vi "TPM with correction version 10-1-1 imaging.vi"() -> ()   [LabVIEW 2012]
uses:
  <vilib>/_Imagine Optic/VIs drivers/Data Haso/Wavefront parameters.ctl
  Program Files/Imagine Optic/Casao LabVIEW SDK/Casao/Casao/Loop prefs.ctl
  <vilib>/_Imagine Optic/VIs drivers/Data Haso/DataHaso.ctl
  <vilib>/Utility/file.llb/Read From Spreadsheet File (DBL).vi
  <vilib>/Utility/file.llb/Write To Spreadsheet File (DBL).vi
panel:
  in  "galvo phase":dbl=89.0
  out "output path":path
  out "Model Coefficients (µm) after":sgl[](array[numeric])
  out "Model Coefficients (µm) before":sgl[](array[numeric])
  in  "stop":bool
  out "Slice now":dbl
  in  "Iteration #":u16(ring)=1 items=["1"=1, "2"=2, "3"=3, "4"=4, "5"=5]
  in  "AO Exp Time":dbl(ring)=0.5 items=["0.2s"=0.2, "0.5s"=0.5, "1.0s"=1.0, "1.5s"=1.5]
  out "after correction":T1
  in  "Filter y tilt":bool=TRUE
  in  "Filter x tilt":bool=TRUE
  in  "Curvature filter":bool=TRUE
  out "PV":dbl
  out "RMS":dbl
  in  "Matrix path":path=path "C:/Documents and Settings/User/Desktop/zw/20160113 200nm bead command matrix.aomc"
  in  "Offset path":path=path "C:/Documents and Settings/User/Desktop/zw/2016-02-09 system resolution/100nm bead correction.dat"
  out "Camera image":u32[][](graph)
  out "RMS":dbl
  out "PV":dbl
  out "before correction":T1
  in  "Curvature filter":bool=TRUE
  in  "Filter y tilt":bool=TRUE
  in  "Filter x tilt":bool=TRUE
  out "after correction":dbl[][](graph) caption="Wavefront"
  out "before correction":dbl[][](graph) caption="Wavefront"
  in  "EMCCD ImExp Time (s)":dbl(ring)=0.5 items=["0.2"=0.2, "0.5"=0.5, "1.0"=1.0, "4.0"=4.0, "8.0"=8.0]
  in  "Step size(um)":dbl
  in  "Laser Power%(0-100)":dbl=10.0
  in  "Slices #":dbl=1.0
  in  "Average Frame #":dbl=10.0
  in  "Correction":bool
  # "OFF"
  # "ON"
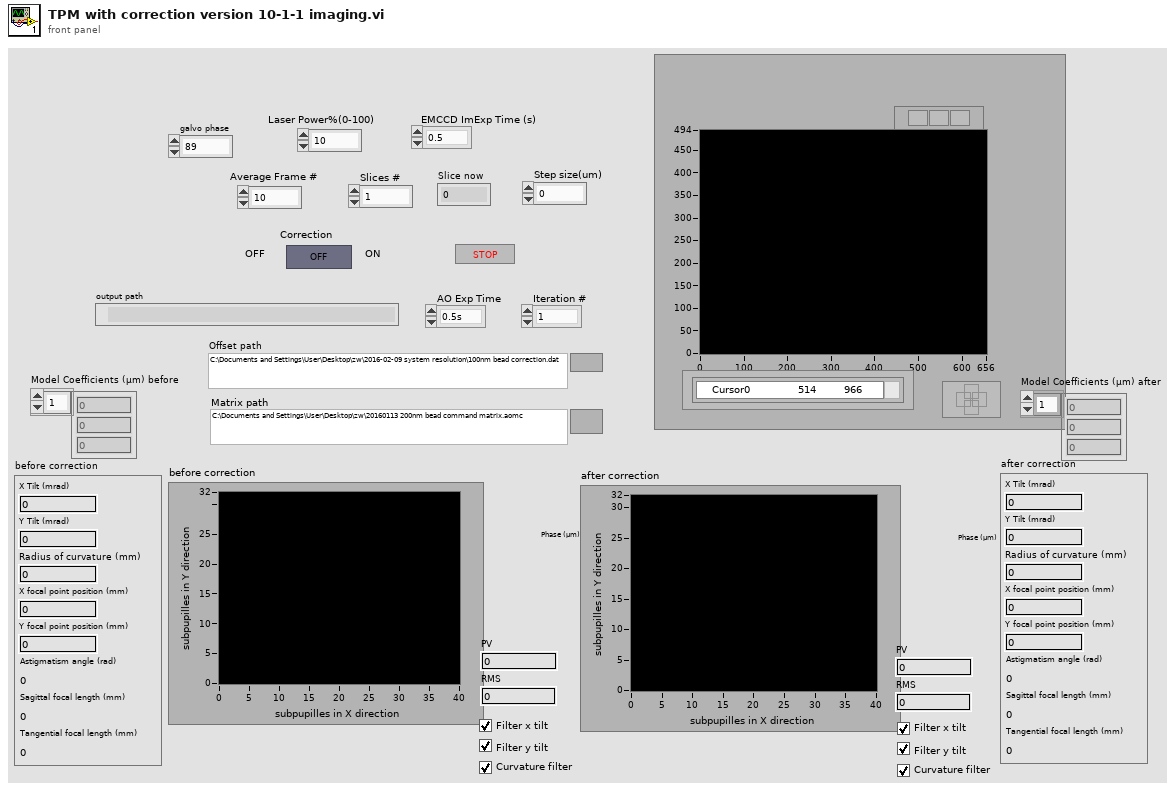
[diagram p1: front panel]
types:
  T1 = typedef "Wavefront parameters.ctl" = cluster{"X Tilt (mrad)":sgl, "Y Tilt (mrad)":sgl, "Radius of curvature (mm)":sgl, "X focal point position (mm)":sgl, "Y focal point position (mm)":sgl, "Astigmatism angle (rad)":sgl, "Sagittal focal length (mm)":sgl, "Tangential focal length (mm)":sgl}
  T2 = typedef "Loop prefs.ctl" = cluster{"Filter tilt on measurement (closed loop)":bool, "Correction gain (closed loop)":sgl, "Limit of subapertures off in CGP (%)":sgl, "Limit of saturated actuators (%)":sgl}
  T3 = cluster{"Filtre tilt X":bool, "Filtre tilt Y":bool, "Filtre courbure":bool}
  T4 = typedef "DataHaso.ctl" = i32
  T5 = cluster{"Measurement":T4, "Target":T4, "Manual target":T4}
  T6 = cluster{"Target for tilt":T4, "Target for focus":T4, "Target for all other aberrations":T4}
  T7 = typedef "Camera.ctl" = i32
  T8 = typedef "PhaseModul.ctl" = i32
  T9 = typedef "Haso.ctl" = i32
  T10 = typedef "Casao.ctl" = i32
  T11 = typedef "Image Compat.ctl" = cluster{"Signed/unsigned":bool, "Number of bits":T12, "Internal object id":i32, "Internal data id":i32}
  T12 = typedef "Data alignment enum.ctl" = enum16{"8", "16", "32"}
  T13 = typedef "Reconstruction prefs.ctl" = cluster{"Reconstruction type":enum16{"Modal", "Zonal"}, "Polynomial type":enum16{"Zernike", "Legendre"}, "Modal reconstruction prefs":T14, "Zonal reconstruction prefs":T17}
  T14 = typedef "Modal reconstruction prefs.ctl" = cluster{"Number of coefficients":u32, "Filtered coefficients":u32[], "RMS Zernike normalization":bool, "Matrix inversion method":u16, "Add zonal residual to modal fit ":bool, "Detection prefs":T15}
  T15 = typedef "PupilDetectionPrefs.ctl" = cluster{"Automatic pupil detection":bool, "Central occultation pupil":bool, "Semi-automatic pupil detection (find radius)":bool, "Semi-automatic pupil detection (find center)":bool, "Automatic pupil detection mode":enum16{"Contained", "Containing"}, "Start coordinates":cluster{"Pupil center (Zernike)":T16, "Pupil radius (Zernike)":sgl, "Pupil center (Legendre)":T16, "Pupil halfsize (Legendre)":T16}}
  T16 = typedef "Point2Df.ctl" = cluster{"X":sgl, "Y":sgl}
  T17 = typedef "Zonal reconstruction prefs.ctl" = cluster{"Number of weak iterations":u16, "Number of max iterations":u32, "Residual limit":sgl}
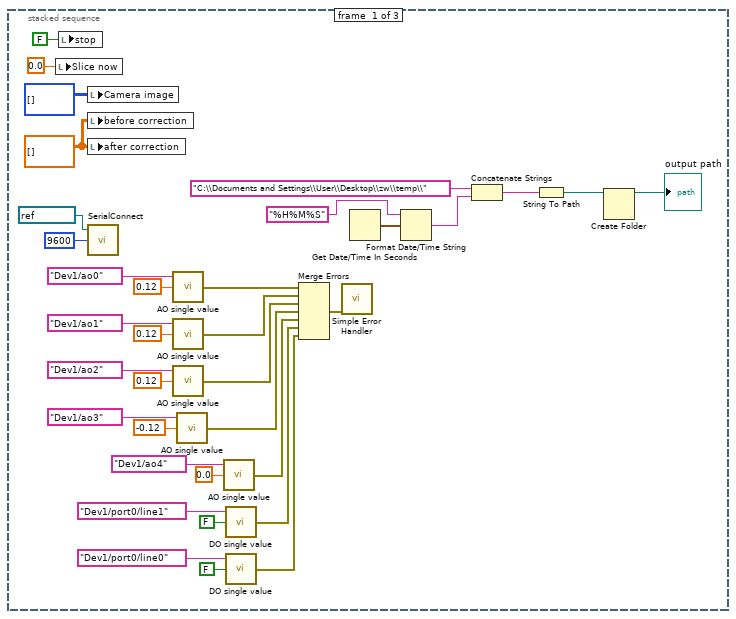
[diagram p2: hidden frame]
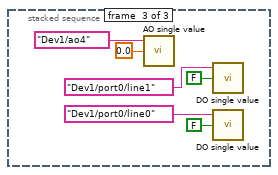
[diagram p10: hidden frame]
diagram:
  n1 = stacked-sequence {
    frame #0 {
      w34 = dbl[][] [] ("before correction")
      n2 = local write "Slice now"(0.0 ("Slice now")) -> ()
      n3 = local write "stop"(FALSE ("stop")) -> ()
      n4 = local write "Camera image"(u32[][] [] ("Camera image")) -> ()
      n5 = local write "before correction"(w34) -> ()
      n6 = local write "after correction"(w34) -> ()
      n7 = call "SerialConnect.vi"("baud rate (9600)"=u32 9600, "VISA resource name"=refnum<visa-resource-name> "COM1") -> ()  [unwired: 1 in, 3 out]
      n8 = call "AO single value.vi"("data"=0.12, "physical channels"=tag "Dev1/ao0") -> ("error out"=w17:errorcluster)  [unwired: 1 in]
      n9 = call "AO single value.vi"("data"=0.12, "physical channels"=tag "Dev1/ao1") -> ("error out"=w16:errorcluster)  [unwired: 1 in]
      n10 = call "AO single value.vi"("data"=0.12, "physical channels"=tag "Dev1/ao2") -> ("error out"=w15:errorcluster)  [unwired: 1 in]
      n11 = call "AO single value.vi"("data"=-0.12, "physical channels"=tag "Dev1/ao3") -> ("error out"=w14:errorcluster)  [unwired: 1 in]
      n12 = call "AO single value.vi"("data"=0.0, "physical channels"=tag "Dev1/ao4") -> ("error out"=w13:errorcluster)  [unwired: 1 in]
      n13 = call "DO single value.vi"("data"=FALSE, "lines"=tag "Dev1/port0/line1") -> ("error out"=w12:errorcluster)  [unwired: 1 in]
      n14 = call "DO single value.vi"("data"=FALSE, "lines"=tag "Dev1/port0/line0") -> ("error out"=w10:errorcluster)  [unwired: 1 in]
      n15 = Merge Errors(w17, w16, w15, w14, w13, w12, w10) -> (w11:errorcluster)
      n16 = call <vilib>:"Simple Error Handler.vi"("error in (no error)"=w11) -> ()  [unwired: 4 in, 5 out]
      n17 = Get Date/Time In Seconds() -> (seconds since 1Jan1904=w2:timestamp)
      n18 = Format Date/Time String(time format string (%c)="%H%M%S", seconds (now)=w2) -> (date/time string=w5:string)  [unwired: 1 in]
      n19 = Concatenate Strings("C:\\Documents and Settings\\User\\Desktop\\zw\\temp\\" ("string"), w5) -> (w6:string)
      n20 = String To Path(string=w6) -> (path=w7:path)
      n21 = Create Folder(path (use dialog)=w7) -> (created path=→"output path":path)  [unwired: 2 in, 2 out]
    }
    frame #1 {
      n22 = case shown="False" "Correction" {
        frame False {
          n23 = flat-sequence {
            frame #0 {
              n24 = call "DO single value.vi"("data"=TRUE, "lines"=tag "Dev1/port0/line1") -> ()  [unwired: 1 in, 1 out]
              n25 = call "DO single value.vi"("data"=FALSE, "lines"=tag "Dev1/port0/line0") -> ()  [unwired: 1 in, 1 out]
            }
            frame #1 {
              n26 = for {
                N: "Slices #" -> [_]
                i -> [w45]
                n27 = local read "stop"() -> (w43:bool)
                n28 = Not(x=w43) -> (.not. x?=w42:bool)
                n29 = Increment(x=w45) -> (x+1=w44:i32)
                n30 = case shown="True" w42 {
                  tunnel: w44 -> [_ w46]
                  frame False {
                  }
                  frame True {
                    n31 = flat-sequence {
                      frame #0 {
                        n32 = for {
                          N: "Average Frame #" -> [_]
                          n33 = local read "stop"() -> (w48:bool)
                          n34 = Not(x=w48) -> (.not. x?=w49:bool)
                          n35 = case shown="True" w49 {
                            frame False {
                            }
                            frame True {
                              n36 = flat-sequence {
                                tunnel: [w52] -> w50
                                tunnel: w50 -> [w74]
                                frame #0 {
                                n37 = local read "Laser Power%(0-100)"() -> (w63:dbl)
                                n38 = local read "EMCCD ImExp Time (s)"() -> (w62:dbl)
                                n39 = local read "galvo phase"() -> (w51:dbl)
                                n40 = call "waveform gen.vi"("Boolean"=TRUE, "galvo phase"=w51, "Exposure Time (s)"=w62, "Laser Power%(0-100)"=w63) -> ("waveform"=w60:waveform(dbl)[])
                                n41 = Index Array(array=w60, index=4) -> (element=w61:waveform(dbl))
                                n42 = call "AO triggle.vi"("physical channels"=tag "Dev1/ao0:4", "data"=w60, "waveform"=w61, "trig source"=tag "/Dev1/PFI1") -> ("task out"=w57:refnum<k21>, "error out"=w54:errorcluster)  [unwired: 1 in]
                                n43 = call "DO single value.vi"("error in"=w54, "data"=TRUE, "lines"=tag "Dev1/port0/line0") -> ("error out"=w53:errorcluster)
                                n44 = while {
                                tunnel: [w72] -> w66
                                tunnel: [w71] -> w65
                                tunnel: w57 -> [w69]
                                tunnel: w53 -> [w68]
                                stop <- w70 stop-if-true
                                n45 = call <vilib>:"DAQmx Is Task Done.vi"("task/channels in"=w69, "error in"=w68) -> ("task out"=w72:refnum<k21>, "task done?"=w70:bool, "error out"=w71:errorcluster)  [unwired: 11 in]
                                }
                                n46 = call <vilib>:"DAQmx Clear Task.vi"("task in"=w66, "error in"=w65) -> ("error out"=w52:errorcluster)  [unwired: 13 in]
                                }
                                frame #1 {
                                n47 = call "DO single value.vi"("error in"=w74, "data"=FALSE, "lines"=tag "Dev1/port0/line0") -> ("error out"=w73:errorcluster)
                                n48 = call "AO single value.vi"("error in"=w73, "data"=0.0, "physical channels"=tag "Dev1/ao4") -> ()  [unwired: 1 out]
                                }
                              }
                            }
                          }
                        }
                      }
                      frame #1 {
                        n49 = local read "Step size(um)"() -> (w79:dbl)
                        n50 = Multiply(x=w79, y=10.0) -> (x*y=w81:dbl)
                        n51 = Number To Decimal String(number=w81) -> (decimal integer string=w84:string)  [unwired: 1 in]
                        n52 = Concatenate Strings("movrel z=", w84) -> (w83:string)
                        n53 = call "WriteCmd.vi"("Command"=w83, "VISA resource name"=refnum<visa-resource-name> "COM1") -> ()  [unwired: 1 in, 1 out]
                      }
                      frame #2 {
                        n54 = Wait (ms)(milliseconds to wait=u32 50) -> ()  [unwired: 1 out]
                      }
                    }
                    n55 = local write "Slice now"(w46) -> ()
                  }
                }
              }
            }
            frame #2 {
            }
          }
        }
        frame True {
          n56 = flat-sequence {
            tunnel: [w102] -> w94
            tunnel: [w104] -> w93
            tunnel: [w103] -> w92
            tunnel: [w102] -> w91
            tunnel: [w101] -> w90
            tunnel: [w100] -> w88
            tunnel: [w95] -> w87
            tunnel: w94 -> [w123]
            tunnel: w93 -> [w122]
            tunnel: w92 -> [w121]
            tunnel: w91 -> [w118]
            tunnel: w90 -> [w117]
            tunnel: [w120] -> w89
            tunnel: w88 -> [w114]
            tunnel: w87 -> [w115]
            tunnel: w89 -> [w638]
            frame #0 {
              n57 = call "AO single value.vi"("data"=0.0, "physical channels"=tag "Dev1/ao4") -> ()  [unwired: 1 in, 1 out]
              n58 = local read "AO Exp Time"() -> (w105:dbl)
              n59 = call-poly <vilib>:"Read From Spreadsheet File.vi"("format (%.3f)"="%.8f", "file path (dialog if empty)"="Offset path") -> ("first row"=w95:dbl[])  [unwired: 5 in, 4 out]
              n60 = call "DO single value.vi"("data"=TRUE, "lines"=tag "Dev1/port0/line1") -> ()  [unwired: 1 in, 1 out]
              n61 = call "DO single value.vi"("data"=FALSE, "lines"=tag "Dev1/port0/line0") -> ()  [unwired: 1 in, 1 out]
              n62 = call "AO init.vi"("Exposure duration specified (s)"=w105, "Commands in"=w95, "Matrix path"="Matrix path") -> ("error out"=w102:errorcluster, "Camera"=w104:T7, "Mirror"=w100:T8, "Haso"=w103:T9, "Casao"=w101:T10)  [unwired: 3 in, 1 out]
            }
            frame #1 {
              n63 = call "Casao Set Preferences.vi"("error in (no error)"=w118, "Loop preferences"=T2 {"Filter tilt on measurement (closed loop)"=FALSE, "Correction gain (closed loop)"=0.75, "Limit of subapertures off in CGP (%)"=0.0, "Limit of saturated actuators (%)"=0.0}, "Casao"=w117) -> ("error out"=w112:errorcluster, "Casao (dup)"=w116:T10)  [unwired: 3 in]
              n64 = local read "Slices #"() -> (w124:dbl)
              n65 = call "PhaseModul apply command.vi"("error in (no error)"=w112, "Commands in"=w115, "Mirror"=w114) -> ("error out"=w111:errorcluster, "Mirror (dup)"=w113:T8)  [unwired: 2 in, 1 out]
              n66 = for {
                N: w124 -> [_]
                tunnel: w123 -> [w138]
                tunnel: w122 -> [w137]
                tunnel: w121 -> [w136]
                tunnel: w111 -> [w126]
                tunnel: [w135] -> w120
                tunnel: w113 -> [w127]
                tunnel: w116 -> [w134]
                tunnel: w115 -> [w125]
                i -> [w130]
                n67 = local read "stop"() -> (w132:bool)
                n68 = Increment(x=w130) -> (x+1=w133:i32)
                n69 = local write "Slice now"(w133) -> ()
                n70 = Not(x=w132) -> (.not. x?=w131:bool)
                n71 = case shown="True" w131 {
                  tunnel: w138 -> [_ w147]
                  tunnel: w137 -> [_ w146]
                  tunnel: w136 -> [_ w145]
                  tunnel: w126 -> [_ w144]
                  tunnel: [w139 w141] -> w135
                  tunnel: w127 -> [_ w143]
                  tunnel: w134 -> [w139 w142]
                  tunnel: w125 -> [_ w140]
                  frame False {
                  }
                  frame True {
                    n72 = flat-sequence {
                      tunnel: w147 -> [w187]
                      tunnel: w146 -> [w186]
                      tunnel: w145 -> [w185]
                      tunnel: w144 -> [w181]
                      tunnel: w143 -> [w172]
                      tunnel: w142 -> [w170]
                      tunnel: [w149] -> w141
                      tunnel: w140 -> [w148]
                      frame #0 {
                        n73 = flat-sequence {
                          tunnel: w170 -> [w190]
                          tunnel: w172 -> [w191]
                          tunnel: w181 -> [w192]
                          tunnel: w185 -> [w193]
                          tunnel: w186 -> [w194]
                          tunnel: w187 -> [w195]
                          tunnel: [w195] -> w155
                          tunnel: [w194] -> w154
                          tunnel: [w193] -> w153
                          tunnel: [w192] -> w152
                          tunnel: [w191] -> w151
                          tunnel: [w190] -> w150
                          tunnel: [w202] -> w161
                          tunnel: [w201] -> w160
                          tunnel: [w200] -> w159
                          tunnel: [w199] -> w158
                          tunnel: [w198] -> w157
                          tunnel: [w197] -> w156
                          tunnel: w155 -> [w202]
                          tunnel: w154 -> [w201]
                          tunnel: w153 -> [w200]
                          tunnel: w152 -> [w199]
                          tunnel: w151 -> [w198]
                          tunnel: w150 -> [w197]
                          tunnel: [w231] -> w184
                          tunnel: [w240] -> w183
                          tunnel: [w239] -> w182
                          tunnel: [w235] -> w180
                          tunnel: [w236] -> w179
                          tunnel: [w233] -> w173
                          tunnel: w161 -> [w232]
                          tunnel: w160 -> [w240]
                          tunnel: w159 -> [w239]
                          tunnel: w158 -> [w236]
                          tunnel: w157 -> [w234]
                          tunnel: w156 -> [w235]
                          tunnel: w148 -> [w230]
                          tunnel: w184 -> [w282]
                          tunnel: w183 -> [w281]
                          tunnel: w182 -> [w280]
                          tunnel: w180 -> [w279]
                          tunnel: w179 -> [w278]
                          tunnel: [w258] -> w178
                          tunnel: [w257] -> w177
                          tunnel: [w253] -> w176
                          tunnel: [w251] -> w175
                          tunnel: [w249] -> w174
                          tunnel: w173 -> [w244]
                          tunnel: [w243] -> w171
                          tunnel: [w241] -> w163
                          tunnel: w178 -> [w424]
                          tunnel: w177 -> [w423]
                          tunnel: w176 -> [w421]
                          tunnel: w175 -> [w420]
                          tunnel: w174 -> [w419]
                          tunnel: [w418] -> w169
                          tunnel: w171 -> [w417]
                          tunnel: [w416] -> w168
                          tunnel: [w415] -> w167
                          tunnel: [w414] -> w166
                          tunnel: [w413] -> w165
                          tunnel: [w412] -> w164
                          tunnel: w163 -> [w411]
                          tunnel: [w411] -> w162
                          tunnel: w169 -> [w603]
                          tunnel: w168 -> [w622]
                          tunnel: w167 -> [w621]
                          tunnel: w166 -> [w620]
                          tunnel: w165 -> [w610]
                          tunnel: w164 -> [w611]
                          tunnel: w162 -> [w609]
                          tunnel: [w603] -> w149
                          frame #0 {
                            n74 = call "AO single value.vi"("data"=-5.0, "physical channels"=tag "Dev1/ao5") -> ()  [unwired: 1 in, 1 out]
                          }
                          frame #1 {
                            n75 = local read "Average Frame #"() -> (w196:dbl)
                            n76 = for {
                              N: w196 -> [_]
                              n77 = local read "stop"() -> (w203:bool)
                              n78 = Not(x=w203) -> (.not. x?=w204:bool)
                              n79 = case shown="True" w204 {
                                frame False {
                                }
                                frame True {
                                n80 = flat-sequence {
                                frame #0 {
                                n81 = local read "Laser Power%(0-100)"() -> (w216:dbl)
                                n82 = local read "EMCCD ImExp Time (s)"() -> (w215:dbl)
                                n83 = call "waveform gen.vi"("Boolean"=TRUE, "galvo phase"="galvo phase", "Exposure Time (s)"=w215, "Laser Power%(0-100)"=w216) -> ("waveform"=w213:waveform(dbl)[])
                                n84 = Index Array(array=w213, index=4) -> (element=w214:waveform(dbl))
                                n85 = call "AO triggle.vi"("physical channels"=tag "Dev1/ao0:4", "data"=w213, "waveform"=w214, "trig source"=tag "/Dev1/PFI0") -> ("task out"=w210:refnum<k21>, "error out"=w207:errorcluster)  [unwired: 1 in]
                                n86 = call "DO single value.vi"("error in"=w207, "data"=TRUE, "lines"=tag "Dev1/port0/line0") -> ("error out"=w206:errorcluster)
                                n87 = while {
                                tunnel: [w225] -> w219
                                tunnel: [w224] -> w218
                                tunnel: w210 -> [w222]
                                tunnel: w206 -> [w221]
                                stop <- w223 stop-if-true
                                n88 = call <vilib>:"DAQmx Is Task Done.vi"("task/channels in"=w222, "error in"=w221) -> ("task out"=w225:refnum<k21>, "task done?"=w223:bool, "error out"=w224:errorcluster)  [unwired: 11 in]
                                }
                                n89 = call <vilib>:"DAQmx Clear Task.vi"("task in"=w219, "error in"=w218) -> ()  [unwired: 13 in, 1 out]
                                }
                                frame #1 {
                                n90 = call "AO single value.vi"("data"=0.0, "physical channels"=tag "Dev1/ao4") -> ()  [unwired: 1 in, 1 out]
                                n91 = call "DO single value.vi"("data"=FALSE, "lines"=tag "Dev1/port0/line0") -> ()  [unwired: 1 in, 1 out]
                                }
                                }
                                }
                              }
                            }
                          }
                          frame #2 {
                            n92 = call "PhaseModul apply command.vi"("error in (no error)"=w232, "Commands in"=w230, "Mirror"=w234) -> ("error out"=w231:errorcluster, "Mirror (dup)"=w233:T8)  [unwired: 2 in, 1 out]
                            n93 = call "AO single value.vi"("data"=1.0, "physical channels"=tag "Dev1/ao5") -> ()  [unwired: 1 in, 1 out]
                          }
                          frame #3 {
                            n94 = flat-sequence {
                              tunnel: [w291] -> w277
                              tunnel: [w290] -> w276
                              tunnel: [w289] -> w275
                              tunnel: [w288] -> w274
                              tunnel: [w287] -> w273
                              tunnel: w280 -> [w289]
                              tunnel: w281 -> [w290]
                              tunnel: w282 -> [w291]
                              tunnel: [w286] -> w272
                              tunnel: w279 -> [w286]
                              tunnel: [w285] -> w271
                              tunnel: w278 -> [w285]
                              tunnel: [w284] -> w245
                              tunnel: w244 -> [w284]
                              tunnel: w277 -> [w307]
                              tunnel: w276 -> [w308]
                              tunnel: w275 -> [w309]
                              tunnel: [w309] -> w270
                              tunnel: [w306] -> w269
                              tunnel: [w305] -> w268
                              tunnel: [w304] -> w267
                              tunnel: w274 -> [w304]
                              tunnel: [w303] -> w266
                              tunnel: w273 -> [w303]
                              tunnel: [w302] -> w265
                              tunnel: w272 -> [w302]
                              tunnel: [w301] -> w264
                              tunnel: w271 -> [w301]
                              tunnel: [w300] -> w246
                              tunnel: w245 -> [w300]
                              tunnel: w270 -> [w321]
                              tunnel: [w321] -> w261
                              tunnel: [w320] -> w262
                              tunnel: w269 -> [w320]
                              tunnel: [w319] -> w263
                              tunnel: w268 -> [w319]
                              tunnel: w267 -> [w314]
                              tunnel: w266 -> [w313]
                              tunnel: [w312] -> w260
                              tunnel: w265 -> [w312]
                              tunnel: [w311] -> w259
                              tunnel: w264 -> [w311]
                              tunnel: [w310] -> w247
                              tunnel: w246 -> [w310]
                              tunnel: w263 -> [w403]
                              tunnel: w262 -> [w363]
                              tunnel: w261 -> [w364]
                              tunnel: w260 -> [w389]
                              tunnel: w259 -> [w388]
                              tunnel: [w367] -> w256
                              tunnel: [w366] -> w255
                              tunnel: [w365] -> w254
                              tunnel: [w364] -> w252
                              tunnel: [w363] -> w250
                              tunnel: [w362] -> w248
                              tunnel: w247 -> [w361]
                              tunnel: [w361] -> w242
                              tunnel: [w335] -> w241
                              tunnel: [w409] -> w257
                              tunnel: [w410] -> w258
                              tunnel: w256 -> [w410]
                              tunnel: w255 -> [w409]
                              tunnel: w254 -> [w408]
                              tunnel: [w407] -> w253
                              tunnel: w252 -> [w407]
                              tunnel: [w406] -> w251
                              tunnel: w250 -> [w406]
                              tunnel: [w405] -> w249
                              tunnel: w248 -> [w405]
                              tunnel: [w404] -> w243
                              tunnel: w242 -> [w404]
                              frame #0 {
                                n95 = local read "Laser Power%(0-100)"() -> (w297:dbl)
                                n96 = local read "AO Exp Time"() -> (w296:dbl)
                                n97 = local read "galvo phase"() -> (w283:dbl)
                                n98 = call "waveform gen.vi"("Boolean"=FALSE, "galvo phase"=w283, "Exposure Time (s)"=w296, "Laser Power%(0-100)"=w297) -> ("waveform"=w295:waveform(dbl)[])
                                n99 = Index Array(array=w295, index=4) -> (element=w294:waveform(dbl))
                                n100 = call "AO triggle.vi"("physical channels"=tag "Dev1/ao0:4", "data"=w295, "waveform"=w294, "trig source"=tag "/Dev1/PFI1") -> ("task out"=w288:refnum<k21>, "error out"=w287:errorcluster)  [unwired: 1 in]
                              }
                              frame #1 {
                                n101 = call <vilib>:"Camera Start.vi"("error in (no error)"=w307, "camera"=w308) -> ("error out"=w305:errorcluster, "camera (dup)"=w306:T7)  [unwired: 4 in]
                              }
                              frame #2 {
                                n102 = while {
                                tunnel: [w326] -> w316
                                tunnel: [w325] -> w315
                                tunnel: w314 -> [w323]
                                tunnel: w313 -> [w322]
                                stop <- w324 stop-if-true
                                n103 = call <vilib>:"DAQmx Is Task Done.vi"("task/channels in"=w323, "error in"=w322) -> ("task out"=w326:refnum<k21>, "task done?"=w324:bool, "error out"=w325:errorcluster)  [unwired: 11 in]
                                }
                                n104 = call "DO single value.vi"("data"=TRUE, "lines"=tag "Dev1/port0/line0") -> ()  [unwired: 1 in, 1 out]
                                n105 = call <vilib>:"DAQmx Clear Task.vi"("task in"=w316, "error in"=w315) -> ()  [unwired: 13 in, 1 out]
                              }
                              frame #3 {
                                n106 = call <vilib>:"Camera Get image.vi"("error in (no error)"=w403, "camera"=w363) -> ("error out"=w385:errorcluster, "Image"=w386:T11, "camera (dup)"=w387:T7)  [unwired: 3 in]
                                n107 = call <vilib>:"Camera Stop.vi"("error in (no error)"=w385, "camera"=w387) -> ()  [unwired: 4 in, 2 out]
                                n108 = call "Image get data.vi"("error in (no error)"=w385, "Image Compat"=w386) -> ("error out"=w375:errorcluster, "Array"=w384:u32[][], "Image Compat (dup)"=w374:T11)  [unwired: 3 in]
                                n109 = call "AO single value.vi"("data"=0.0, "physical channels"=tag "Dev1/ao4") -> ()  [unwired: 1 in, 1 out]
                                n110 = local write "Camera image"(w384) -> ()
                                n111 = call <vilib>:"Haso compute slopes.vi"("error in (no error)"=w375, "Image Compat"=w374, "Haso"=w364) -> ("error out"=w333:errorcluster, "Data Haso"=w337:T4)  [unwired: 1 in, 2 out]
                                n112 = call "DO single value.vi"("data"=FALSE, "lines"=tag "Dev1/port0/line0") -> ()  [unwired: 1 in, 1 out]
                                n113 = call "DataHaso ctor copie.vi"("error in (no error)"=w333, "DataHaso"=w337) -> ("error out"=w332:errorcluster, "new DataHaso"=w335:T4, "DataHaso (dup)"=w334:T4)  [unwired: 3 in]
                                n114 = call "DataHaso get reconstruction prefs.vi"("error in (no error)"=w332, "Data Haso"=w334) -> ("error out"=w348:errorcluster, "Reconstruction Preferences"=w344:T13, "Data Haso (dup)"=w347:T4)  [unwired: 3 in]
                                n115 = Bundle By Name(cluster=w344, "Reconstruction type"=enum16{"Modal", "Zonal"}."Modal", "Polynomial type"=enum16{"Zernike", "Legendre"}."Zernike", "Modal reconstruction prefs.Number of coefficients"=u32 32) -> (w343:T13)
                                n116 = call <vilib>:"DataHaso set reconstruction prefs.vi"("error in (no error)"=w348, "Reconstruction Preferences"=w343, "Data Haso"=w347) -> ("error out"=w345:errorcluster, "Data Haso (dup)"=w346:T4)  [unwired: 3 in]
                                n117 = call "DataHaso get modal coefficients.vi"("error in (no error)"=w345, "Data Haso"=w346) -> ("error out"=w338:errorcluster, "Coefficients (µm)"=w349:sgl[], "Data Haso (dup)"=w339:T4)  [unwired: 3 in]
                                "Model Coefficients (µm) before" <- w349
                                n118 = Bundle By Name(cluster=T3 {"Filtre tilt X"=FALSE, "Filtre tilt Y"=FALSE, "Filtre courbure"=FALSE} ("Filtre"), "Filtre tilt X"="Filter x tilt", "Filtre tilt Y"="Filter y tilt", "Filtre courbure"="Curvature filter") -> (w369:T3)
                                n119 = call <vilib>:"DataHaso parameters.vi"("error in (no error)"=w338, "Data Haso"=w339) -> ("error out"=w382:errorcluster, "Parameters"=w357:T1, "Data Haso (dup)"=w383:T4)  [unwired: 3 in]
                                "before correction" <- w357
                                n120 = control-ref of="before correction"() -> (w368:refnum<vi>)
                                n121 = call "DataHaso filter tilt or curvature.vi"("error in (no error)"=w382, "Filter (default: all true)"=w369, "Data Haso"=w383) -> ("error out"=w380:errorcluster, "Data Haso (dup)"=w381:T4)  [unwired: 3 in]
                                n122 = local read "Slice now"() -> (w351:dbl)
                                n123 = call "DataHaso phase.vi"("error in (no error)"=w380, "Data Haso"=w381) -> ("error out"=w378:errorcluster, "Phase (µm)"=w379:i32, "Data Haso (dup)"=w336:T4)  [unwired: 3 in]
                                n124 = Number To Decimal String(number=w351) -> (decimal integer string=w353:string)  [unwired: 1 in]
                                n125 = call "Formatter Intensity Graph.vi"("error in (no error)"=w378, "Intensity Graph"=w368, "Surface with pupil"=w379) -> ("error out"=w376:errorcluster, "Surface with pupil (dup)"=w377:i32)  [unwired: 2 in, 1 out]
                                n126 = call <vilib>:"Surface with pupil get stats.vi"("error in (no error)"=w376, "Surface Avec Pupille"=w377) -> ("error out"=w362:errorcluster, "PV"=w360:sgl, "RMS"=w359:dbl)  [unwired: 2 in, 1 out]
                                "PV" <- w360
                                "RMS" <- w359
                                n127 = local read "output path"() -> (w327:path)
                                n128 = Concatenate Strings("before_slice", w353, ".dat") -> (w328:string)
                                n129 = Cluster To Array(cluster=w357) -> (array=w358:sgl[])
                                n130 = Build Path(base path=w327, name or relative path=w328) -> (appended path=w329:path)
                                n131 = Build Array (concatenate)(w360, w359, w358, w349) -> (w356:dbl[])
                                n132 = Merge Errors(w362, w388) -> (w398:errorcluster)
                                n133 = Bundle By Name(cluster=T6 {"Target for tilt"=0, "Target for focus"=0, "Target for all other aberrations"=0} ("References"), "Target for tilt"=w335, "Target for focus"=w335) -> (w401:T6)
                                n134 = call "DataHaso ctor copie.vi"("error in (no error)"=w398, "DataHaso"=w336) -> ("error out"=w400:errorcluster, "new DataHaso"=w399:T4)  [unwired: 3 in, 1 out]
                                n135 = call-poly <vilib>:"Write To Spreadsheet File.vi"("transpose? (no:F)"=TRUE, "format (%.3f)"="%.6f", "1D data"=w356, "file path (dialog if empty)"=w329) -> ()  [unwired: 4 in, 1 out]
                                n136 = call "Casao Compute target.vi"("error in (no error)"=w400, "Targets"=w401, "DataHaso"=w399, "Casao"=w389) -> ("error out"=w396:errorcluster, "DataHaso (dup)"=w365:T4, "Casao (dup)"=w397:T10)  [unwired: 1 out]
                                n137 = Bundle By Name(cluster=T5 {"Measurement"=0, "Target"=0, "Manual target"=0} ("Slopes"), "Measurement"=w336, "Target"=w365) -> (w395:T5)
                                n138 = call "Casao get correction commands.vi"("Casao"=w397, "Slopes"=w395, "error in (no error)"=w396) -> ("Casao (dup)"=w367:T10, "Commands"=w392:sgl[], "error out"=w393:errorcluster)  [unwired: 2 in, 2 out]
                                n139 = call "PhaseModul apply command.vi"("error in (no error)"=w393, "Commands in"=w392, "Mirror"=w361) -> ("error out"=w366:errorcluster)  [unwired: 2 in, 2 out]
                              }
                              frame #4 {
                                n140 = call "DataHaso dtor.vi"("Data Haso"=w408) -> ()  [unwired: 6 in, 1 out]
                              }
                            }
                          }
                          frame #4 {
                            n141 = for {
                              N: "Iteration #" -> [_]
                              tunnel: w424 -> [w453]
                              tunnel: w423 -> [w452]
                              tunnel: w421 -> [w451]
                              tunnel: w420 -> [w450]
                              tunnel: w419 -> [w449]
                              tunnel: [w447] -> w418
                              tunnel: w417 -> [w442]
                              tunnel: [w441] -> w416
                              tunnel: [w439] -> w415
                              tunnel: [w437] -> w414
                              tunnel: [w435] -> w413
                              tunnel: [w432] -> w412
                              tunnel: w411 -> [w431]
                              i -> [w430]
                              n142 = Increment(x=w430) -> (x+1=w429:i32)
                              n143 = flat-sequence {
                                tunnel: [w478] -> w472
                                tunnel: [w479] -> w471
                                tunnel: [w480] -> w470
                                tunnel: [w484] -> w469
                                tunnel: [w483] -> w468
                                tunnel: [w482] -> w467
                                tunnel: [w481] -> w466
                                tunnel: w453 -> [w482]
                                tunnel: w452 -> [w481]
                                tunnel: w451 -> [w480]
                                tunnel: w450 -> [w479]
                                tunnel: w449 -> [w478]
                                tunnel: [w477] -> w443
                                tunnel: w442 -> [w477]
                                tunnel: w429 -> [w475]
                                tunnel: [w474] -> w426
                                tunnel: w472 -> [w501]
                                tunnel: w471 -> [w502]
                                tunnel: w470 -> [w503]
                                tunnel: [w503] -> w465
                                tunnel: [w500] -> w464
                                tunnel: [w499] -> w463
                                tunnel: [w498] -> w462
                                tunnel: w469 -> [w498]
                                tunnel: [w497] -> w461
                                tunnel: w468 -> [w497]
                                tunnel: [w496] -> w460
                                tunnel: w467 -> [w496]
                                tunnel: [w495] -> w459
                                tunnel: w466 -> [w495]
                                tunnel: [w494] -> w444
                                tunnel: w443 -> [w494]
                                tunnel: [w493] -> w427
                                tunnel: w426 -> [w493]
                                tunnel: w465 -> [w516]
                                tunnel: [w516] -> w456
                                tunnel: [w515] -> w457
                                tunnel: w464 -> [w515]
                                tunnel: [w514] -> w458
                                tunnel: w463 -> [w514]
                                tunnel: w462 -> [w509]
                                tunnel: w461 -> [w508]
                                tunnel: [w507] -> w455
                                tunnel: w460 -> [w507]
                                tunnel: [w506] -> w454
                                tunnel: w459 -> [w506]
                                tunnel: [w505] -> w445
                                tunnel: w444 -> [w505]
                                tunnel: [w504] -> w428
                                tunnel: w427 -> [w504]
                                tunnel: w458 -> [w584]
                                tunnel: w457 -> [w585]
                                tunnel: w456 -> [w586]
                                tunnel: w455 -> [w571]
                                tunnel: w454 -> [w570]
                                tunnel: [w550] -> w448
                                tunnel: [w549] -> w446
                                tunnel: w445 -> [w529]
                                tunnel: [w545] -> w440
                                tunnel: [w544] -> w438
                                tunnel: [w543] -> w436
                                tunnel: [w542] -> w434
                                tunnel: [w531] -> w433
                                tunnel: w431 -> [w528]
                                tunnel: w428 -> [w525]
                                tunnel: [w522] -> w425
                                tunnel: w448 -> [w598]
                                tunnel: [w597] -> w447
                                tunnel: w446 -> [w597]
                                tunnel: [w596] -> w441
                                tunnel: w440 -> [w596]
                                tunnel: [w595] -> w439
                                tunnel: w438 -> [w595]
                                tunnel: [w594] -> w437
                                tunnel: w436 -> [w594]
                                tunnel: [w590] -> w435
                                tunnel: w434 -> [w591]
                                tunnel: w433 -> [w593]
                                tunnel: [w593] -> w432
                                tunnel: w425 -> [w592]
                                frame #0 {
                                n144 = local read "Laser Power%(0-100)"() -> (w490:dbl)
                                n145 = local read "AO Exp Time"() -> (w489:dbl)
                                n146 = local read "galvo phase"() -> (w473:dbl)
                                n147 = call "waveform gen.vi"("Boolean"=FALSE, "galvo phase"=w473, "Exposure Time (s)"=w489, "Laser Power%(0-100)"=w490) -> ("waveform"=w488:waveform(dbl)[])
                                n148 = local read "Iteration #"() -> (w476:u16)
                                n149 = Index Array(array=w488, index=4) -> (element=w487:waveform(dbl))
                                n150 = Less?(x=w476, y=w475) -> (x < y?=w474:bool)
                                n151 = call "AO triggle.vi"("physical channels"=tag "Dev1/ao0:4", "data"=w488, "waveform"=w487, "trig source"=tag "/Dev1/PFI1") -> ("task out"=w484:refnum<k21>, "error out"=w483:errorcluster)  [unwired: 1 in]
                                }
                                frame #1 {
                                n152 = call <vilib>:"Camera Start.vi"("error in (no error)"=w501, "camera"=w502) -> ("error out"=w499:errorcluster, "camera (dup)"=w500:T7)  [unwired: 4 in]
                                }
                                frame #2 {
                                n153 = while {
                                tunnel: [w521] -> w511
                                tunnel: [w520] -> w510
                                tunnel: w509 -> [w518]
                                tunnel: w508 -> [w517]
                                stop <- w519 stop-if-true
                                n154 = call <vilib>:"DAQmx Is Task Done.vi"("task/channels in"=w518, "error in"=w517) -> ("task out"=w521:refnum<k21>, "task done?"=w519:bool, "error out"=w520:errorcluster)  [unwired: 11 in]
                                }
                                n155 = call "DO single value.vi"("data"=TRUE, "lines"=tag "Dev1/port0/line0") -> ()  [unwired: 1 in, 1 out]
                                n156 = call <vilib>:"DAQmx Clear Task.vi"("task in"=w511, "error in"=w510) -> ()  [unwired: 13 in, 1 out]
                                }
                                frame #3 {
                                n157 = call <vilib>:"Camera Get image.vi"("error in (no error)"=w584, "camera"=w585) -> ("error out"=w567:errorcluster, "Image"=w568:T11, "camera (dup)"=w569:T7)  [unwired: 3 in]
                                n158 = call <vilib>:"Camera Stop.vi"("error in (no error)"=w567, "camera"=w569) -> ()  [unwired: 4 in, 2 out]
                                n159 = call "Image get data.vi"("error in (no error)"=w567, "Image Compat"=w568) -> ("error out"=w557:errorcluster, "Array"=w566:u32[][], "Image Compat (dup)"=w556:T11)  [unwired: 3 in]
                                n160 = call "AO single value.vi"("data"=0.0, "physical channels"=tag "Dev1/ao4") -> ()  [unwired: 1 in, 1 out]
                                n161 = local write "Camera image"(w566) -> ()
                                n162 = call <vilib>:"Haso compute slopes.vi"("error in (no error)"=w557, "Image Compat"=w556, "Haso"=w586) -> ("error out"=w534:errorcluster, "Data Haso"=w533:T4)  [unwired: 1 in, 2 out]
                                n163 = call "DO single value.vi"("data"=FALSE, "lines"=tag "Dev1/port0/line0") -> ()  [unwired: 1 in, 1 out]
                                n164 = call "DataHaso get reconstruction prefs.vi"("error in (no error)"=w534, "Data Haso"=w533) -> ("error out"=w540:errorcluster, "Reconstruction Preferences"=w539:T13, "Data Haso (dup)"=w541:T4)  [unwired: 3 in]
                                n165 = Bundle By Name(cluster=w539, "Reconstruction type"=enum16{"Modal", "Zonal"}."Modal", "Polynomial type"=enum16{"Zernike", "Legendre"}."Zernike", "Modal reconstruction prefs.Number of coefficients"=u32 32) -> (w538:T13)
                                n166 = call <vilib>:"DataHaso set reconstruction prefs.vi"("error in (no error)"=w540, "Reconstruction Preferences"=w538, "Data Haso"=w541) -> ("error out"=w526:errorcluster, "Data Haso (dup)"=w527:T4)  [unwired: 3 in]
                                n167 = call "DataHaso get modal coefficients.vi"("error in (no error)"=w526, "Data Haso"=w527) -> ("error out"=w532:errorcluster, "Coefficients (µm)"=w531:sgl[], "Data Haso (dup)"=w530:T4)  [unwired: 3 in]
                                "Model Coefficients (µm) after" <- w531
                                n168 = Bundle By Name(cluster=T3 {"Filtre tilt X"=FALSE, "Filtre tilt Y"=FALSE, "Filtre courbure"=FALSE} ("Filtre"), "Filtre tilt X"="Filter x tilt", "Filtre tilt Y"="Filter y tilt", "Filtre courbure"="Curvature filter") -> (w554:T3)
                                n169 = call <vilib>:"DataHaso parameters.vi"("error in (no error)"=w532, "Data Haso"=w530) -> ("error out"=w564:errorcluster, "Parameters"=w543:T1, "Data Haso (dup)"=w565:T4)  [unwired: 3 in]
                                "after correction" <- w543
                                n170 = control-ref of="after correction"() -> (w548:refnum<vi>)
                                n171 = call "DataHaso filter tilt or curvature.vi"("error in (no error)"=w564, "Filter (default: all true)"=w554, "Data Haso"=w565) -> ("error out"=w562:errorcluster, "Data Haso (dup)"=w563:T4)  [unwired: 3 in]
                                n172 = call "DataHaso phase.vi"("error in (no error)"=w562, "Data Haso"=w563) -> ("error out"=w560:errorcluster, "Phase (µm)"=w561:i32, "Data Haso (dup)"=w547:T4)  [unwired: 3 in]
                                n173 = call "Formatter Intensity Graph.vi"("error in (no error)"=w560, "Intensity Graph"=w548, "Surface with pupil"=w561) -> ("error out"=w558:errorcluster, "Surface with pupil (dup)"=w559:i32)  [unwired: 2 in, 1 out]
                                n174 = call <vilib>:"Surface with pupil get stats.vi"("error in (no error)"=w558, "Surface Avec Pupille"=w559) -> ("error out"=w579:errorcluster, "PV"=w544:sgl, "RMS"=w545:dbl)  [unwired: 2 in, 1 out]
                                "RMS" <- w545
                                "PV" <- w544
                                n175 = Merge Errors(w579, w570) -> (w578:errorcluster)
                                n176 = Bundle By Name(cluster=T6 {"Target for tilt"=0, "Target for focus"=0, "Target for all other aberrations"=0} ("References"), "Target for tilt"=w528, "Target for focus"=w528) -> (w582:T6)
                                n177 = call "DataHaso ctor copie.vi"("error in (no error)"=w578, "DataHaso"=w547) -> ("error out"=w581:errorcluster, "new DataHaso"=w580:T4, "DataHaso (dup)"=w546:T4)  [unwired: 3 in]
                                n178 = call "Casao Compute target.vi"("error in (no error)"=w581, "Targets"=w582, "DataHaso"=w580, "Casao"=w571) -> ("error out"=w576:errorcluster, "DataHaso (dup)"=w550:T4, "Casao (dup)"=w577:T10)  [unwired: 1 out]
                                n179 = Bundle By Name(cluster=T5 {"Measurement"=0, "Target"=0, "Manual target"=0} ("Slopes"), "Measurement"=w546, "Target"=w550) -> (w575:T5)
                                n180 = call "Casao get correction commands.vi"("Casao"=w577, "Slopes"=w575, "error in (no error)"=w576) -> ("Casao (dup)"=w549:T10, "Commands"=w542:sgl[], "error out"=w522:errorcluster)  [unwired: 2 in, 2 out]
                                n181 = case shown="True" w525 {
                                tunnel: w522 -> [_ w589]
                                tunnel: w542 -> [_ w588]
                                tunnel: w529 -> [_ w587]
                                frame False {
                                }
                                frame True {
                                n182 = call "PhaseModul apply command.vi"("error in (no error)"=w589, "Commands in"=w588, "Mirror"=w587) -> ()  [unwired: 2 in, 3 out]
                                }
                                }
                                }
                                frame #4 {
                                n183 = call "DataHaso dtor.vi"("Data Haso"=w598) -> ()  [unwired: 6 in, 1 out]
                                n184 = case shown="Error" w592 {
                                tunnel: w591 -> [w599 _]
                                tunnel: [w599 w600] -> w590
                                frame No Error {
                                }
                                frame Error {
                                n185 = Initialize Array(0.0 ("element"), 52 ("dimension size")) -> (w600:dbl[])
                                }
                                }
                                }
                              }
                            }
                          }
                          frame #5 {
                            n186 = call "DataHaso dtor.vi"("Data Haso"=w609) -> ()  [unwired: 6 in, 1 out]
                            n187 = local read "Slice now"() -> (w614:dbl)
                            n188 = Cluster To Array(cluster=w620) -> (array=w619:sgl[])
                            n189 = Build Array (concatenate)(w621, w622, w619, w611) -> (w627:dbl[])
                            n190 = Number To Decimal String(number=w614) -> (decimal integer string=w624:string)  [unwired: 1 in]
                            n191 = Number To Decimal String(number=w614) -> (decimal integer string=w616:string)  [unwired: 1 in]
                            n192 = call "AO single value.vi"("data"=0.0, "physical channels"=tag "Dev1/ao4") -> ()  [unwired: 1 in, 1 out]
                            n193 = local read "output path"() -> (w604:path)
                            n194 = Concatenate Strings("afterC_slice", w624, ".dat") -> (w608:string)
                            n195 = Concatenate Strings("command", w616, ".dat") -> (w605:string)
                            n196 = Build Path(base path=w604, name or relative path=w608) -> (appended path=w607:path)
                            n197 = Build Path(base path=w604, name or relative path=w605) -> (appended path=w606:path)
                            n198 = call-poly <vilib>:"Write To Spreadsheet File.vi"("transpose? (no:F)"=TRUE, "format (%.3f)"="%.6f", "1D data"=w627, "file path (dialog if empty)"=w607) -> ()  [unwired: 4 in, 1 out]
                            n199 = call-poly <vilib>:"Write To Spreadsheet File.vi"("transpose? (no:F)"=TRUE, "format (%.3f)"="%.6f", "1D data"=w610, "file path (dialog if empty)"=w606) -> ()  [unwired: 4 in, 1 out]
                          }
                          frame #6 {
                            n200 = local read "Step size(um)"() -> (w636:dbl)
                            n201 = Multiply(x=w636, y=10.0) -> (x*y=w634:dbl)
                            n202 = Number To Decimal String(number=w634) -> (decimal integer string=w631:string)  [unwired: 1 in]
                            n203 = Concatenate Strings("movrel z=", w631) -> (w632:string)
                            n204 = call "WriteCmd.vi"("Command"=w632, "VISA resource name"=refnum<visa-resource-name> "COM1") -> ()  [unwired: 1 in, 1 out]
                          }
                          frame #7 {
                            n205 = Wait (ms)(milliseconds to wait=u32 50) -> ()  [unwired: 1 out]
                          }
                        }
                      }
                    }
                  }
                }
                n206 = call "AO single value.vi"("data"=0.0, "physical channels"=tag "Dev1/ao4") -> ()  [unwired: 1 in, 1 out]
              }
            }
            frame #2 {
              n207 = call "Casao dtor.vi"("Casao"=w638) -> ()  [unwired: 6 in, 1 out]
            }
          }
        }
      }
    }
    frame #2 {
      n208 = call "AO single value.vi"("data"=0.0, "physical channels"=tag "Dev1/ao4") -> ()  [unwired: 1 in, 1 out]
      n209 = call "DO single value.vi"("data"=FALSE, "lines"=tag "Dev1/port0/line1") -> ()  [unwired: 1 in, 1 out]
      n210 = call "DO single value.vi"("data"=FALSE, "lines"=tag "Dev1/port0/line0") -> ()  [unwired: 1 in, 1 out]
    }
  }
